vi "AMZ_S3_APIHLP_Parse PUT Object Request Parameters.vi"(7 "PUT Object Request Parameters":T1={"Content Type"="binary/octet-stream", "ACL"=enum."private", "Storage Class"=enum."STANDARD", "User Metadata"=[], "Content MD5"=""}, 8 "error in (no error)":errorcluster, 11 "HTTP Headers in":T5[](array[typedef])) -> (0 "error out":errorcluster, 3 "HTTP Headers":T5[](array[typedef]))   [LabVIEW 2015, in "LV Interface for Amazon S3.lvlib"]
uses:
  LV Interface for Amazon S3.lvlib
  Typedefs/AMZ_S3_HTTP Header-Value pair.ctl
  Typedefs/AMZ_S3_API_PUT Object Request Parameters.ctl
  Typedefs/AMZ_S3_ACL.ctl
  Typedefs/AMZ_S3_Storage Class.ctl
  Typedefs/AMZ_S3_Object Metadata.ctl
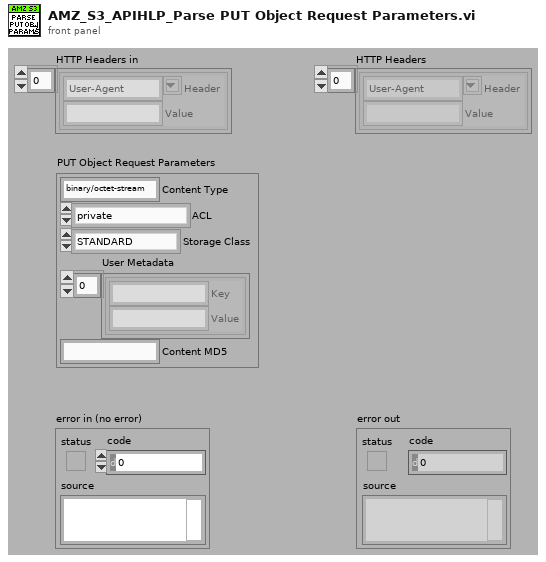
[diagram p1: front panel]
types:
  T1 = typedef "LV Interface for Amazon S3.lvlib/AMZ_S3_API_PUT Object Request Parameters.ctl" = cluster{"Content Type":string, "ACL":T2, "Storage Class":T3, "User Metadata":T4[], "Content MD5":string}
  T2 = typedef "LV Interface for Amazon S3.lvlib/AMZ_S3_ACL.ctl" = enum16{"private", "public-read", "public-read-write", "aws-exec-read", "authenticated-read", "bucket-owner-read", "bucket-owner-full-control"}
  T3 = typedef "LV Interface for Amazon S3.lvlib/AMZ_S3_Storage Class.ctl" = enum16{"STANDARD", "REDUCED_REDUNDANCY"}
  T4 = typedef "LV Interface for Amazon S3.lvlib/AMZ_S3_Object Metadata.ctl" = cluster{"Key":string, "Value":string}
  T5 = typedef "LV Interface for Amazon S3.lvlib/AMZ_S3_HTTP Header-Value pair.ctl" = cluster{"Header":string, "Value":string}
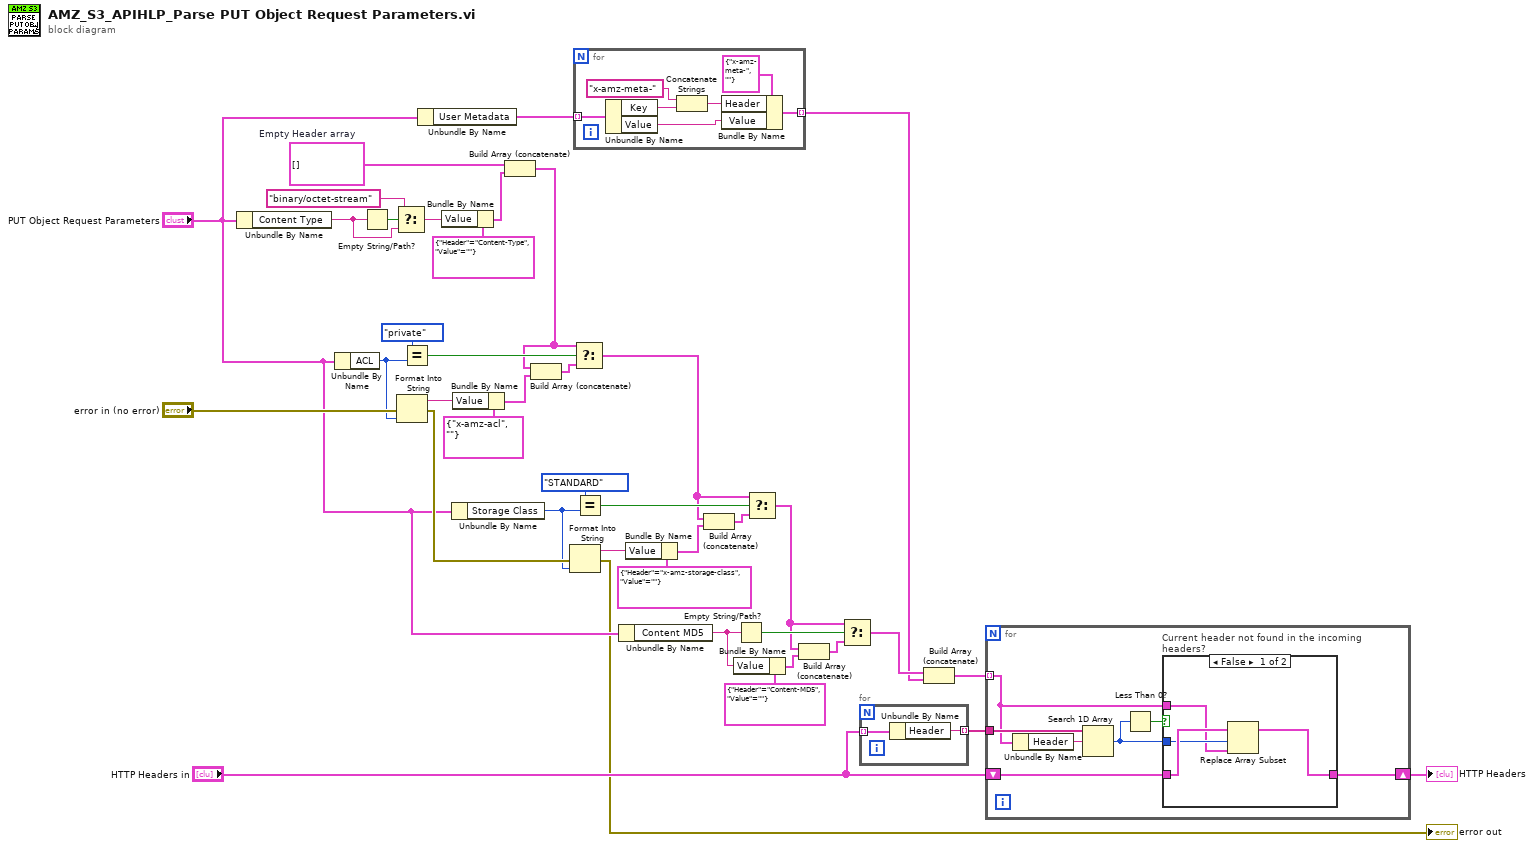
[diagram p0: block diagram]
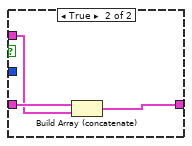
[diagram p2: hidden frame]
diagram:
  w4 = T5[] []  # Empty Header array
  n1 = Unbundle By Name("PUT Object Request Parameters") -> ("Content Type"=w6:string)
  n2 = Unbundle By Name("PUT Object Request Parameters") -> ("ACL"=w34:T2)
  n3 = Empty String/Path?(string/path=w6) -> (empty?=w39:bool)
  n4 = Select(t="binary/octet-stream", s=w39, f=w6) -> (s? t:f=w3:string)
  n5 = Format Into String(error in="error in (no error)", w34) -> (resulting string=w32:string, error out=w23:errorcluster)  [unwired: 2 in]
  n6 = Equal?(x=AMZ_S3_ACL."private", y=w34) -> (x = y?=w37:bool)
  n7 = Unbundle By Name("PUT Object Request Parameters") -> ("User Metadata"=w14:T4[])
  n8 = Bundle By Name(cluster=T5 {"Header"="Content-Type", "Value"=""} ("HTTP Header-Value pair"), "Value"=w3) -> (w2:T5)
  n9 = Unbundle By Name("PUT Object Request Parameters") -> ("Storage Class"=w22:T3)
  n10 = Bundle By Name(cluster=T5 {"Header"="x-amz-acl", "Value"=""} ("HTTP Header-Value pair"), "Value"=w32) -> (w31:T5)
  n11 = Build Array (concatenate)(w4, w2) -> (w1:T5[])
  n12 = Build Array (concatenate)(w1, w31) -> (w36:T5[])
  n13 = Format Into String(error in=w23, w22) -> (resulting string=w29:string, error out=→"error out":errorcluster)  [unwired: 2 in]
  n14 = for {
    tunnel: w14 -> [w47] mode=indexing
    tunnel: [w41] -> w12 mode=indexing
    n15 = Unbundle By Name(w47) -> ("Key"=w45:string, "Value"=w42:string)
    n16 = Concatenate Strings("x-amz-meta-", w45) -> (w43:string)
    n17 = Bundle By Name(cluster=T5 {"Header"="x-amz-meta-", "Value"=""} ("HTTP Header-Value pair"), "Header"=w43, "Value"=w42) -> (w41:T5)
  }
  n18 = Select(t=w1, s=w37, f=w36) -> (s? t:f=w24:T5[])
  n19 = Equal?(x=AMZ_S3_Storage_Class."STANDARD", y=w22) -> (x = y?=w26:bool)
  n20 = Unbundle By Name("PUT Object Request Parameters") -> ("Content MD5"=w18:string)
  n21 = Bundle By Name(cluster=T5 {"Header"="x-amz-storage-class", "Value"=""} ("HTTP Header-Value pair"), "Value"=w29) -> (w30:T5)
  n22 = Build Array (concatenate)(w24, w30) -> (w27:T5[])
  n23 = Bundle By Name(cluster=T5 {"Header"="Content-MD5", "Value"=""} ("HTTP Header-Value pair"), "Value"=w18) -> (w19:T5)
  n24 = Empty String/Path?(string/path=w18) -> (empty?=w20:bool)
  n25 = Select(t=w24, s=w26, f=w27) -> (s? t:f=w16:T5[])
  n26 = Build Array (concatenate)(w16, w19) -> (w21:T5[])
  n27 = Select(t=w16, s=w20, f=w21) -> (s? t:f=w13:T5[])
  n28 = for {
    tunnel: "HTTP Headers in" -> [w49] mode=indexing
    tunnel: [w48] -> w10 mode=indexing
    n29 = Unbundle By Name(w49) -> ("Header"=w48:string)
  }
  n30 = Build Array (concatenate)(w13, w12) -> (w11:T5[])
  n31 = for {
    tunnel: w11 -> [w52] mode=indexing
    tunnel: w10 -> [w56]
    shift-right: [w50] -> w8
    shift-left: "HTTP Headers in" -> [w51]
    n32 = Unbundle By Name(w52) -> ("Header"=w55:string)
    n33 = Search 1D Array(1D array=w56, element=w55) -> (index of element=w53:i32)  [unwired: 1 in]
    n34 = Less Than 0?(x=w53) -> (x < 0?=w54:bool)
    n35 = case "Current header not found in the incoming headers?" shown="False" w54 {
      tunnel: w53 -> [w59 _]
      tunnel: w52 -> [w58 w62]
      tunnel: w51 -> [w60 w63]
      tunnel: [w57 w61] -> w50
      frame False {
        n36 = Replace Array Subset(array=w60, new element=w58, index=w59) -> (w57:T5[])
      }
      frame True {
        n37 = Build Array (concatenate)(w63, w62) -> (w61:T5[])
      }
    }
  }
  "HTTP Headers" <- w8
